vi "Query IP Setup.vi"(0 "VISA resource name":refnum<visa-resource-name>, 11 "error in (no error)":errorcluster) -> (4 "VISA resource name out":refnum<visa-resource-name>, 6 "IP Setup Mode":u16(ring) items=["Auto", "Manual"], 15 "error out":errorcluster)   [LabVIEW 2020, in "Associated Research 78XX Series.lvlib"]
doc: "Queries the IP Setup Mode configured in the APT 6000 Series Power Source instrument\n\nNote: This setting is supported for <B>Firmware Version 2.0</B> Only"
uses:
  <instrlib>/Associated Research 78XX Series/Associated Research 78XX Series.lvlib
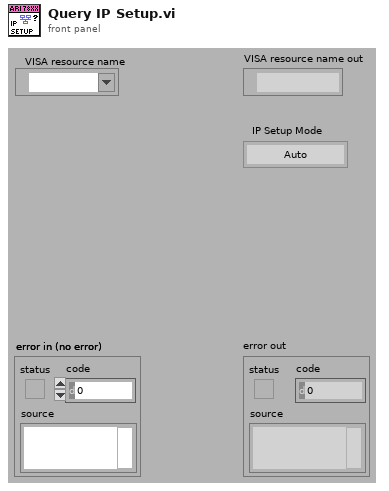
[diagram p1: front panel]
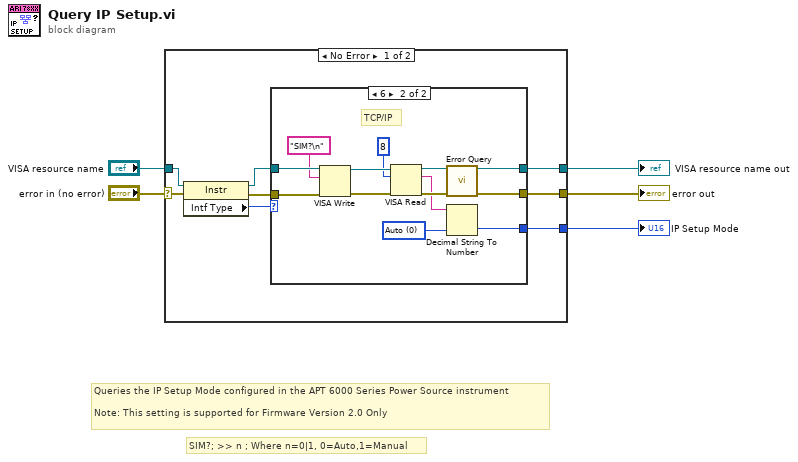
[diagram p0: block diagram]
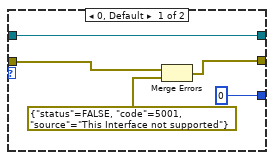
[diagram p2: hidden frame]
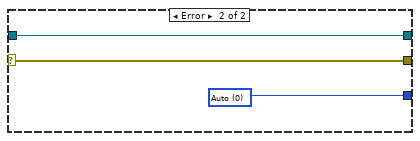
[diagram p3: hidden frame]
diagram:
  # "SIM?; >> n ; Where n=0|1, 0=Auto,1=Manual"
  # "Queries the IP Setup Mode configured in the APT 6000 Series Power Source instrument\n\nNote: This setting is supported for Firmware Version 2.0 Only"
  n1 = case shown="No Error" "error in (no error)" {
    selector: "error in (no error)" -> [w11 w34]
    tunnel: "VISA resource name" -> [w8 w33]
    tunnel: [w13 w33] -> w5
    tunnel: [w12 w34] -> w4
    tunnel: [w10 w32] -> w1
    frame No Error {
      n2 = property class="Instr"(reference=w8, error in=w11) -> (reference out=w7:refnum<visa-resource-name>, error out=w9:errorcluster, "Intf Type"=w6:u16)
      n3 = case shown="6" w6 {
        tunnel: w7 -> [w18 w31]
        tunnel: [w18 w30] -> w13
        tunnel: [w16 w29] -> w12
        tunnel: w9 -> [w15 w27]
        tunnel: [u16 0 w21] -> w10
        frame 0, Default {
          n4 = Merge Errors(w15, errorcluster {"status"=FALSE, "code"=5001, "source"="This Interface not supported"} ("error in 2 (no error)")) -> (w16:errorcluster)
        }
        frame 6 {
          w22 = u16 0 items=["Auto", "Manual"] ("Option")
          # "TCP/IP"
          n5 = VISA Write(VISA resource name=w31, write buffer="SIM?\n" ("Command to Send"), error in (no error)=w27) -> (VISA resource name out=w25:refnum<visa-resource-name>, error out=w26:errorcluster)  [unwired: 1 out]
          n6 = VISA Read(VISA resource name=w25, byte count=u32 8, error in (no error)=w26) -> (VISA resource name out=w24:refnum<visa-resource-name>, read buffer=w19:string, error out=w23:errorcluster)  [unwired: 1 out]
          n7 = call <instrlib>:"Error Query.vi"("VISA resource name"=w24, "error in (no error)"=w23) -> ("VISA resource name out"=w30:refnum<visa-resource-name>, "error out"=w29:errorcluster)  [unwired: 10 in, 2 out]
          n8 = Decimal String To Number(string=w19, default (0L)=w22) -> (number=w21:u16)  [unwired: 1 in, 1 out]
        }
      }
    }
    frame Error {
      w32 = u16 0 items=["Auto", "Manual"] ("Option")
    }
  }
  "error out" <- w4
  "VISA resource name out" <- w5
  "IP Setup Mode" <- w1
